vi "Sequence Macro.vi"(11 "VISA resource name":refnum<visa-resource-name>="COM1") -> (2 "read string":string)   [LabVIEW 2017]
uses:
  controls/#typedef_Macro.ctl
  controls/#typedef_Queue Cmd.ctl
panel:
  out "position":string
  out "status":string
  in  "Array":T1[](array[typedef]) {"Position" max=360 step=1 scale=0.0..360.0}
  in  "Exec Seq Button":bool
  in  "Callib Button":bool
  out "error out":errorcluster
  in  "error in (no error)":errorcluster
  in  "stop":bool
  in  "Get ID Button":bool
  # "Position [deg]"
  # "Speed [tick]"
  # "Wait After [tick]"
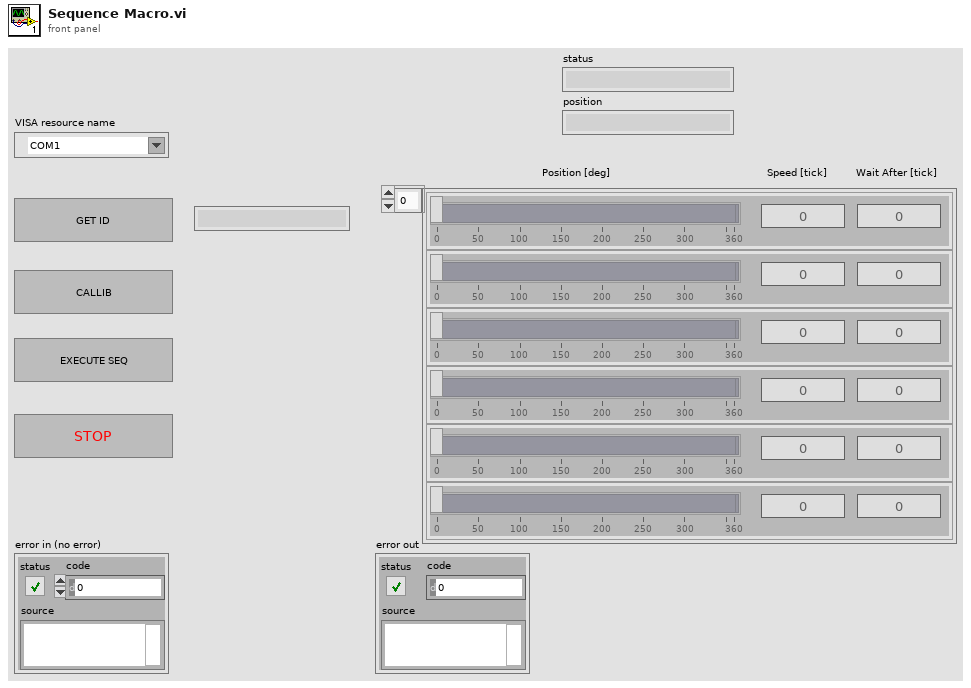
[diagram p1: front panel]
types:
  T1 = typedef "#typedef_Macro.ctl" = cluster{"Position":u16, "Speed":u8, "Wait After":u16}
  T2 = typedef "#typedef_Queue Cmd.ctl" = enum16{"Get ID", "Get Status", "Callib", "GoTo", "GoTo seq", "Macro seq", "Exit"}
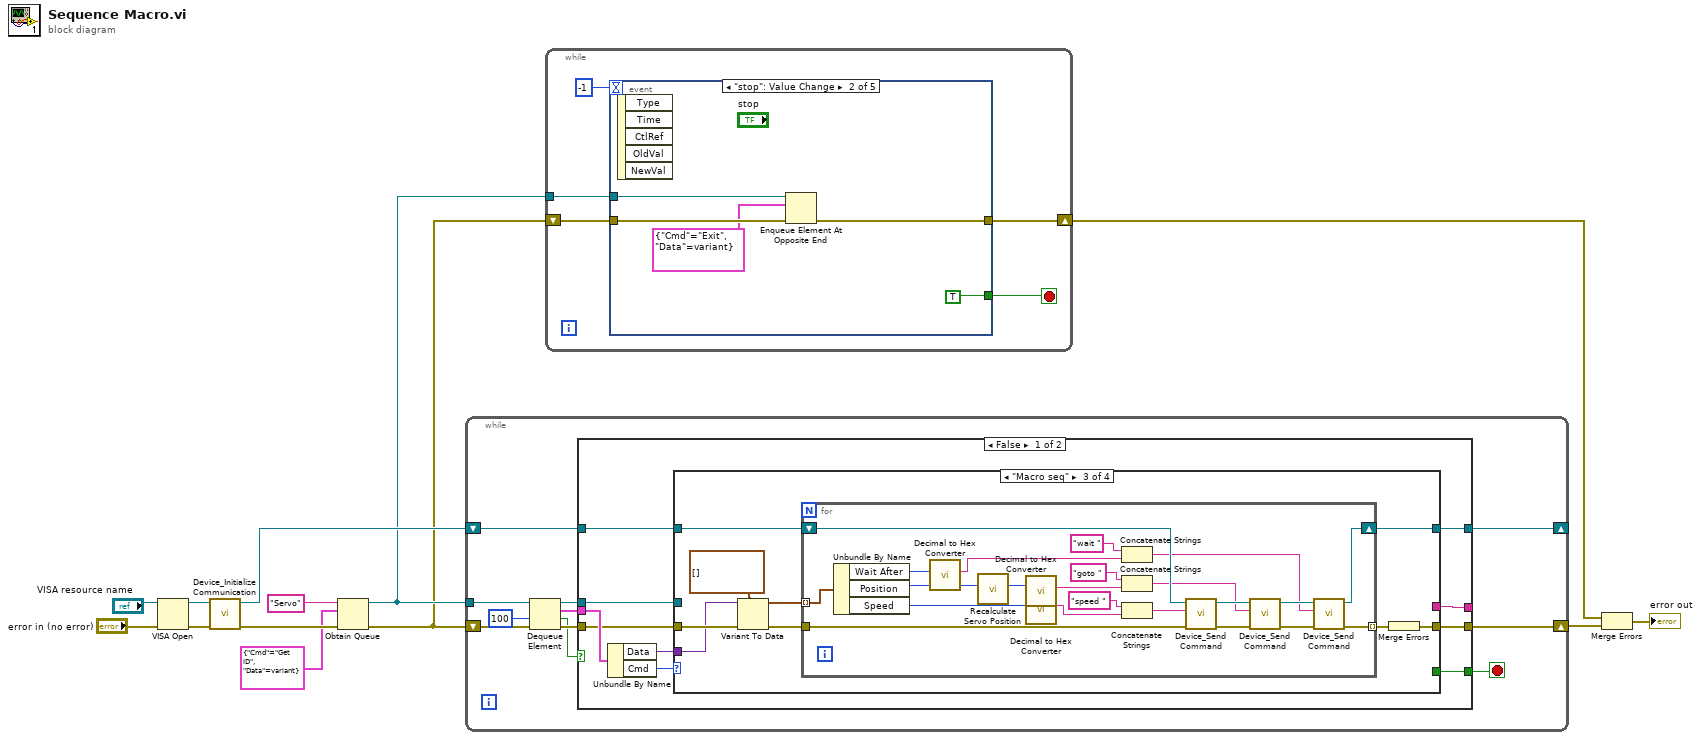
[diagram p0: block diagram]
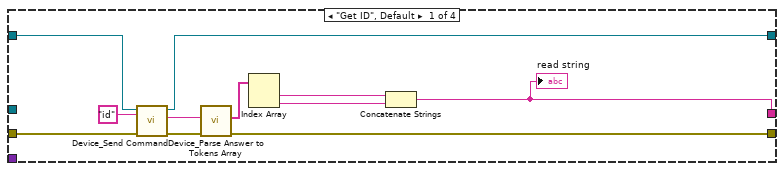
[diagram p2: hidden frame]
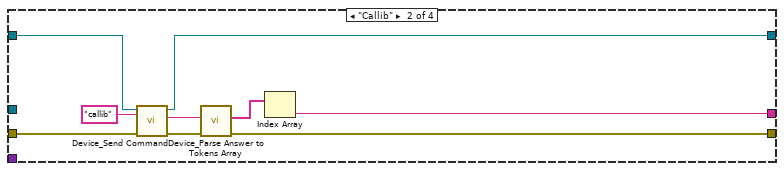
[diagram p3: hidden frame]
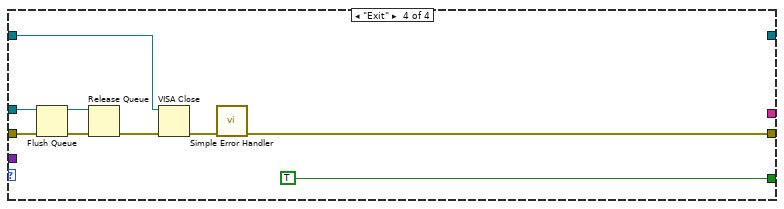
[diagram p4: hidden frame]
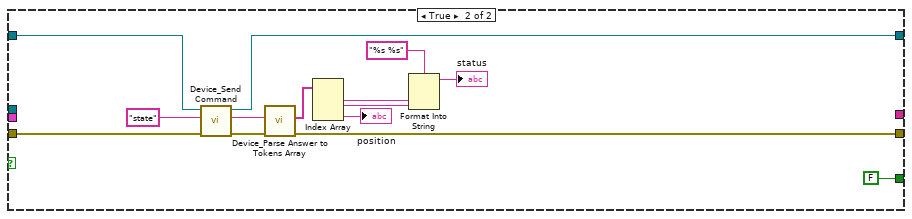
[diagram p5: hidden frame]
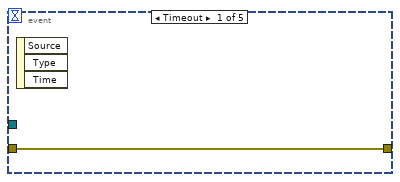
[diagram p6: hidden frame]
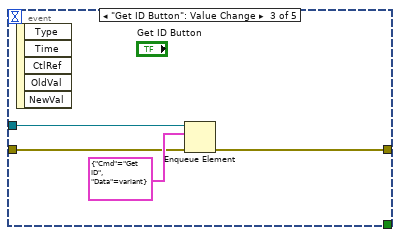
[diagram p7: hidden frame]
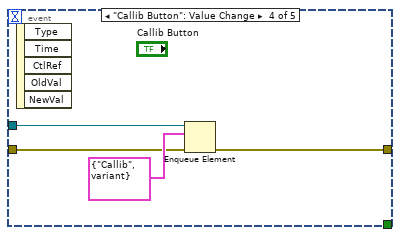
[diagram p8: hidden frame]
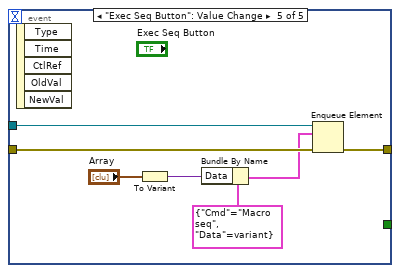
[diagram p9: hidden frame]
diagram:
  n1 = VISA Open(error in (no error)="error in (no error)", VISA resource name="VISA resource name") -> (VISA resource name=w12:refnum<visa-resource-name>, error out=w11:errorcluster)  [unwired: 3 in]
  n2 = call "Device_Initialize Communication.vi"("error in (no error)"=w11, "VISA Refnum in"=w12) -> ("error out"=w9:errorcluster, "VISA Refnum out"=w8:refnum<visa-resource-name>)  [unwired: 8 in]
  n3 = Obtain Queue(name (unnamed)="Servo", element data type=cluster{"Cmd":T2, "Data":variant} {"Cmd"=enum."Get ID", "Data"=variant} ("Queue Msg"), error in (no error)=w9) -> (queue out=w5:refnum<queue>, error out=w4:errorcluster)  [unwired: 2 in, 1 out]
  n4 = while {
    shift-right: [w16] -> _
    shift-left: w8 -> [w17]
    tunnel: w5 -> [w23]
    shift-right: [w19] -> w3
    shift-left: w4 -> [w24]
    stop <- w18 stop-if-true
    n5 = Dequeue Element(queue=w23, timeout in ms (-1)=100, error in (no error)=w24) -> (queue out=w20:refnum<queue>, element=w22:cluster{"Cmd":T2, "Data":variant}, timed out?=w14:bool, error out=w21:errorcluster)
    n6 = case shown="False" w14 {
      tunnel: w22 -> [w34 _]
      tunnel: w21 -> [w32 w108]
      tunnel: w20 -> [w31 _]
      tunnel: [w30 w103] -> w19
      tunnel: [w29 FALSE] -> w18
      tunnel: w17 -> [w28 w107]
      tunnel: [w27 w101] -> w16
      tunnel: [w25 _] -> _
      frame False {
        n7 = Unbundle By Name(w34) -> ("Data"=w26:variant, "Cmd"=w33:T2)
        n8 = case shown="\"Macro seq\"" w33 {
          tunnel: w32 -> [w43 w52 w63 w94]
          tunnel: w31 -> [_ _ _ w87]
          tunnel: [w40 w46 w57 w89] -> w30
          tunnel: [_ _ _ TRUE] -> w29
          tunnel: w28 -> [w44 w53 w55 w91]
          tunnel: [w42 w51 w56 _] -> w27
          tunnel: w26 -> [_ _ w61 _]
          tunnel: [w36 w48 _ _] -> w25
          frame "Get ID", Default {
            n9 = call "Device_Send Command.vi"("error in (no error)"=w43, "write string"="id", "VISA Refnum in"=w44) -> ("error out"=w41:errorcluster, "read buffer"=w39:string, "VISA Refnum out"=w42:refnum<visa-resource-name>)  [unwired: 6 in]
            n10 = call "Device_Parse Answer to Tokens Array.vi"("error in (no error)"=w41, "Answer"=w39) -> ("error out"=w40:errorcluster, "Tokens Array"=w38:string[])  [unwired: 8 in]
            n11 = Index Array(array=w38) -> (element #1=w37:string, element #2=w35:string)  [unwired: 2 in]
            n12 = Concatenate Strings(w37, w35) -> (w36:string)
            "read string" <- w36
          }
          frame "Callib" {
            n13 = call "Device_Send Command.vi"("error in (no error)"=w52, "write string"="callib", "VISA Refnum in"=w53) -> ("error out"=w47:errorcluster, "read buffer"=w49:string, "VISA Refnum out"=w51:refnum<visa-resource-name>)  [unwired: 6 in]
            n14 = call "Device_Parse Answer to Tokens Array.vi"("error in (no error)"=w47, "Answer"=w49) -> ("error out"=w46:errorcluster, "Tokens Array"=w50:string[])  [unwired: 8 in]
            n15 = Index Array(array=w50) -> (element=w48:string)  [unwired: 1 in]
          }
          frame "Macro seq" {
            n16 = Variant To Data(error in=w63, type=T1[] [] ("Array"), Variant=w61) -> (data=w59:T1[], error out=w60:errorcluster)
            n17 = for {
              tunnel: w60 -> [w73]
              tunnel: w59 -> [w85] mode=indexing
              tunnel: [w80] -> w58 mode=indexing
              shift-right: [w76] -> w56
              shift-left: w55 -> [w75]
              n18 = Unbundle By Name(w85) -> ("Wait After"=w84:u16, "Position"=w82:u16, "Speed"=w83:u8)
              n19 = call "Decimal to Hex Converter.vi"("Decimal"=w84) -> ("String"=w65:string)  [unwired: 10 in]
              n20 = call "Recalculate Servo Position.vi"("Position in Degrees"=w82) -> ("Recalculated Position"=w81:u16)  [unwired: 9 in, 1 out]
              n21 = call "Decimal to Hex Converter.vi"("Decimal"=w81) -> ("String"=w68:string)  [unwired: 10 in]
              n22 = call "Decimal to Hex Converter.vi"("Decimal"=w83) -> ("String"=w72:string)  [unwired: 10 in]
              n23 = Concatenate Strings("wait " ("string"), w65) -> (w64:string)
              n24 = Concatenate Strings("goto " ("string"), w68) -> (w67:string)
              n25 = Concatenate Strings("speed " ("string"), w72) -> (w71:string)
              n26 = call "Device_Send Command.vi"("error in (no error)"=w73, "write string"=w71, "VISA Refnum in"=w75) -> ("error out"=w78:errorcluster, "VISA Refnum out"=w74:refnum<visa-resource-name>)  [unwired: 6 in, 1 out]
              n27 = call "Device_Send Command.vi"("error in (no error)"=w78, "write string"=w67, "VISA Refnum in"=w74) -> ("error out"=w79:errorcluster, "VISA Refnum out"=w77:refnum<visa-resource-name>)  [unwired: 6 in, 1 out]
              n28 = call "Device_Send Command.vi"("error in (no error)"=w79, "write string"=w64, "VISA Refnum in"=w77) -> ("error out"=w80:errorcluster, "VISA Refnum out"=w76:refnum<visa-resource-name>)  [unwired: 6 in, 1 out]
            }
            n29 = Merge Errors(w58) -> (w57:errorcluster)
          }
          frame "Exit" {
            n30 = Flush Queue(queue=w87, error in (no error)=w94) -> (queue out=w86:refnum<queue>, error out=w88:errorcluster)  [unwired: 1 out]
            n31 = Release Queue(queue=w86, error in (no error)=w88) -> (error out=w90:errorcluster)  [unwired: 1 in, 2 out]
            n32 = VISA Close(VISA resource name=w91, error in (no error)=w90) -> (error out=w92:errorcluster)
            n33 = call <vilib>:"Simple Error Handler.vi"("error in (no error)"=w92) -> ("error out"=w89:errorcluster)  [unwired: 4 in, 4 out]
          }
        }
      }
      frame True {
        n34 = call "Device_Send Command.vi"("error in (no error)"=w108, "write string"="state", "VISA Refnum in"=w107) -> ("error out"=w104:errorcluster, "read buffer"=w102:string, "VISA Refnum out"=w101:refnum<visa-resource-name>)  [unwired: 6 in]
        n35 = call "Device_Parse Answer to Tokens Array.vi"("error in (no error)"=w104, "Answer"=w102) -> ("error out"=w103:errorcluster, "Tokens Array"=w105:string[])  [unwired: 8 in]
        n36 = Index Array(array=w105) -> (element #1=w98:string, element #2=w97:string, element #3=→"position":string)  [unwired: 3 in]
        n37 = Format Into String(format string="%s %s", w98, w97) -> (resulting string=→"status":string)  [unwired: 2 in, 1 out]
      }
    }
  }
  n38 = while {
    tunnel: w5 -> [w113]
    shift-right: [w111] -> w2
    shift-left: w4 -> [w112]
    stop <- w110 stop-if-true
    n39 = event shown="[1] \"stop\": Value Change" {
      selector: _ -> [_ _ _ _ _]
      dyn-events: _ -> [_ _ _ _ _]
      timeout: -1 -> [_ _ _ _ _]
      tunnel: w113 -> [_ w116 w121 w125 w132]
      tunnel: w112 -> [w114 w119 w122 w126 w133]
      tunnel: [w114 w118 w120 w124 w131] -> w111
      tunnel: [_ TRUE _ _ _] -> w110
      event Timeout {
        n40 = event-data() -> ()  [unwired: 1 in, 3 out]
      }
      event "stop": Value Change {
        n41 = event-data() -> ()  [unwired: 1 in, 5 out]
        n42 = Enqueue Element At Opposite End(queue=w116, element=cluster{"Cmd":T2, "Data":variant} {"Cmd"=enum."Exit", "Data"=variant} ("Queue Msg"), error in (no error)=w119) -> (error out=w118:errorcluster)  [unwired: 1 in, 2 out]
      }
      event "Get ID Button": Value Change {
        n43 = event-data() -> ()  [unwired: 1 in, 5 out]
        n44 = Enqueue Element(queue=w121, element=cluster{"Cmd":T2, "Data":variant} {"Cmd"=enum."Get ID", "Data"=variant} ("Queue Msg"), error in (no error)=w122) -> (error out=w120:errorcluster)  [unwired: 1 in, 2 out]
      }
      event "Callib Button": Value Change {
        n45 = event-data() -> ()  [unwired: 1 in, 5 out]
        n46 = Enqueue Element(queue=w125, element=cluster{"Cmd":T2, "Data":variant} {"Cmd"=enum."Callib", "Data"=variant} ("Queue Msg"), error in (no error)=w126) -> (error out=w124:errorcluster)  [unwired: 1 in, 2 out]
      }
      event "Exec Seq Button": Value Change {
        n47 = event-data() -> ()  [unwired: 1 in, 5 out]
        n48 = To Variant(anything="Array") -> (Variant=w129:variant)
        n49 = Bundle By Name(cluster=cluster{"Cmd":T2, "Data":variant} {"Cmd"=enum."Macro seq", "Data"=variant} ("Queue Msg"), "Data"=w129) -> (w130:cluster{"Cmd":T2, "Data":variant})
        n50 = Enqueue Element(queue=w132, element=w130, error in (no error)=w133) -> (error out=w131:errorcluster)  [unwired: 1 in, 2 out]
      }
    }
  }
  n51 = Merge Errors(w2, w3) -> (→"error out":errorcluster)
